vi "set_H2_0.vi"(0 "Manifold H2 Flow":dbl, 1 "H2 Active":bool, 2 "H2N2 Remote":bool=TRUE) -> ()   [LabVIEW 2011]
uses:
  editor_lib/Flow_Globals.vi
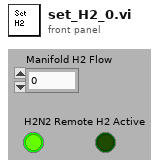
[diagram p1: front panel]
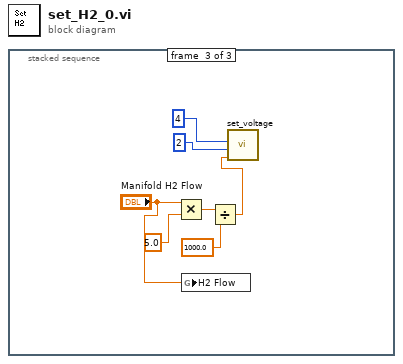
[diagram p0: block diagram]
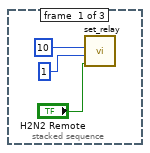
[diagram p2: hidden frame]
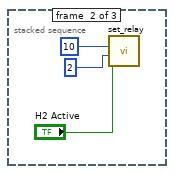
[diagram p3: hidden frame]
diagram:
  n1 = stacked-sequence {
    frame #0 {
      n2 = call "set_relay.vi"("Slot"=10, "Relay"=1, "Relay Status"="H2N2 Remote") -> ()  [unwired: 3 out]
    }
    frame #1 {
      n3 = call "set_relay.vi"("Slot"=10, "Relay"=2, "Relay Status"="H2 Active") -> ()  [unwired: 3 out]
    }
    frame #2 {
      n4 = Multiply(x="Manifold H2 Flow", y=5.0) -> (x*y=w9:dbl)
      n5 = global write "Flow_Globals.vi" "H2 Flow"("Manifold H2 Flow") -> ()
      n6 = Divide(x=w9, y=1000.0) -> (x/y=w11:dbl)
      n7 = call "set_voltage.vi"("Voltage"=w11, "Channel Index"=2 ("Channel"), "Slot"=4) -> ()  [unwired: 1 in, 1 out]
    }
  }
